vi "Main_25A.vi"() -> ()   [LabVIEW 2024]
uses:
  Utility/Universal Utility/TypeDefs_Utility/Cluster_Row-Column.ctl
  9e3f57c0-2ef8-4495-8287-c6a42a5fb955.vi
  Utility/Universal Utility/TypeDefs_Utility/ENUM_4 Directions U-D-L-R.ctl
  Utility/Universal Utility/TypeDefs_Utility/ENUM_8 Directions U-D-L-R.ctl
panel:
  out "Keys":u32[][](array[numeric])
  out "Locks":u32[][](array[numeric])
  in  "Select Data":enum32{"Example", "Puzzle"}(tab)
  in  "Example":string="#####\n.####\n.####\n.####\n.#.#.\n.#...\n.....\n\n#####\n##.##\n.#.##\n...##\n...#.\n...#.\n.....\n\n.....\n#....\n#....\n#...#\n#.#.#\n#.###\n#####\n\n.....\n.....\n#.#..\n###..\n###.#\n###.#\n#####\n\n.....\n.....\n.....\n#....\n#.#..\n#.#.#\n#####"
  in  "Puzzle":string=".....\n..#..\n..#.#\n..#.#\n#.###\n#####\n#####\n\n#####\n.#.##\n.#..#\n.....\n.....\n.....\n.....\n\n.....\n.....\n.....\n....#\n.#.##\n##.##\n#####\n\n.....\n.....\n.....\n#..#.\n#..##\n#.###\n#####\n\n.....\n#....\n#.#..\n###..\n####.\n#####\n#####\n\n.....\n#....\n#....\n#.#.#\n#.#.#\n#.#.#\n#####\n\n#####\n#.#.#\n....#\n....#\n....#\n.....\n.....\n\n#####\n.####\n.##.#\n.##..\n.##..\n..#..\n.....\n\n#####\n#.###\n#.###\n#.###\n#..#.\n.....\n.....\n\n#####\n#.###\n#.###\n#.#.#\n#.#.#\n.....\n.....\n\n.....\n..#..\n#.#..\n###..\n####.\n####.\n#####\n\n.....\n#....\n#.#..\n#.#..\n####.\n####.\n#####\n\n#####\n.###.\n..#..\n..#..\n..#..\n.....\n.....\n\n.....\n....#\n..#.#\n.##.#\n.##.#\n.##.#\n#####\n\n.....\n.....\n..#..\n..##.\n.###.\n.###.\n#####\n\n.....\n.....\n.....\n.#..#\n###.#\n#####\n#####\n\n#####\n##.##\n##.#.\n##.#.\n##...\n.#...\n.....\n\n#####\n#####\n#.###\n#.#.#\n#...#\n#....\n.....\n\n#####\n.#.##\n...##\n....#\n....#\n....#\n.....\n\n.....\n#....\n##..#\n##.##\n##.##\n##.##\n#####\n\n.....\n.....\n#....\n#...#\n#.#.#\n#.#.#\n#####\n\n#####\n.#.##\n.#.#.\n.#...\n.#...\n.#...\n.....\n\n.....\n#....\n##..#\n###.#\n###.#\n###.#\n#####\n\n#####\n###.#\n#.#.#\n#.#.#\n#...#\n#...#\n.....\n\n#####\n##.#.\n##.#.\n.#.#.\n.#...\n.....\n.....\n\n#####\n#####\n.##.#\n.##..\n.#...\n.#...\n.....\n\n#####\n#####\n#.###\n#.###\n#..#.\n#..#.\n.....\n\n.....\n#....\n##...\n##.#.\n####.\n####.\n#####\n\n.....\n....#\n.#.##\n.#.##\n.####\n#####\n#####\n\n.....\n#....\n#.#.#\n#.#.#\n#####\n#####\n#####\n\n#####\n####.\n####.\n#.##.\n..##.\n..#..\n.....\n\n.....\n#....\n##...\n##...\n##.#.\n##.#.\n#####\n\n.....\n.#..#\n.##.#\n.####\n#####\n#####\n#####\n\n.....\n...#.\n...#.\n.#.#.\n#####\n#####\n#####\n\n.....\n.....\n...#.\n..##.\n#.##.\n#####\n#####\n\n#####\n##.#.\n.#.#.\n.#.#.\n.#.#.\n...#.\n.....\n\n#####\n#.#.#\n..#.#\n..#.#\n.....\n.....\n.....\n\n#####\n#####\n.###.\n.###.\n.###.\n.#.#.\n.....\n\n.....\n.....\n..#..\n..#..\n.##.#\n.####\n#####\n\n#####\n#.###\n#.###\n...#.\n...#.\n.....\n.....\n\n.....\n.....\n.#...\n.##..\n.###.\n####.\n#####\n\n.....\n#.#.#\n#.#.#\n###.#\n###.#\n###.#\n#####\n\n#####\n#####\n#####\n#####\n#.##.\n#.#..\n.....\n\n.....\n.....\n..#..\n..#..\n#.#..\n###.#\n#####\n\n#####\n#####\n###.#\n###..\n#.#..\n#.#..\n.....\n\n#####\n#####\n##.##\n#..#.\n#..#.\n#....\n.....\n\n.....\n..#..\n.##..\n###.#\n###.#\n###.#\n#####\n\n.....\n.#...\n.#...\n.#.#.\n.#.##\n.####\n#####\n\n.....\n.#...\n###..\n###.#\n###.#\n###.#\n#####\n\n.....\n...#.\n#.##.\n#####\n#####\n#####\n#####\n\n.....\n...#.\n...#.\n#..#.\n#..#.\n##.#.\n#####\n\n#####\n.####\n.###.\n.#.#.\n.....\n.....\n.....\n\n.....\n#.#..\n#.#.#\n#.###\n#.###\n#####\n#####\n\n#####\n#####\n###.#\n#.#..\n#.#..\n.....\n.....\n\n.....\n#.#..\n#.##.\n####.\n####.\n####.\n#####\n\n#####\n#####\n##.##\n#..#.\n#..#.\n#..#.\n.....\n\n.....\n#.#.#\n#.#.#\n#.#.#\n###.#\n###.#\n#####\n\n#####\n#####\n#####\n####.\n#.##.\n..#..\n.....\n\n.....\n.....\n....#\n....#\n..#.#\n#.#.#\n#####\n\n.....\n..#.#\n#.#.#\n#.#.#\n#.###\n#.###\n#####\n\n#####\n#.##.\n...#.\n...#.\n...#.\n...#.\n.....\n\n.....\n...#.\n.#.##\n#####\n#####\n#####\n#####\n\n#####\n##.##\n##.#.\n##.#.\n#....\n.....\n.....\n\n.....\n..#..\n..#.#\n..###\n.####\n#####\n#####\n\n#####\n####.\n####.\n####.\n##.#.\n.#.#.\n.....\n\n#####\n#####\n###.#\n#.#..\n..#..\n.....\n.....\n\n.....\n#....\n#....\n#...#\n#.#.#\n#.###\n#####\n\n.....\n.....\n#.#.#\n#.#.#\n#.#.#\n#.###\n#####\n\n#####\n.####\n..###\n..#.#\n....#\n.....\n.....\n\n.....\n#...#\n#...#\n#.#.#\n#.#.#\n#.#.#\n#####\n\n#####\n###.#\n###..\n.##..\n..#..\n.....\n.....\n\n.....\n.....\n#..#.\n##.#.\n##.#.\n#####\n#####\n\n.....\n..#..\n..##.\n..##.\n..###\n#.###\n#####\n\n#####\n.##.#\n.#...\n.#...\n.#...\n.#...\n.....\n\n#####\n##.##\n##.##\n.#..#\n.#..#\n.....\n.....\n\n.....\n....#\n#...#\n#...#\n#...#\n#.#.#\n#####\n\n.....\n.....\n#....\n#..#.\n##.#.\n##.##\n#####\n\n.....\n.....\n...#.\n.#.#.\n.#.#.\n####.\n#####\n\n#####\n.####\n..##.\n..##.\n..##.\n...#.\n.....\n\n#####\n#.#.#\n..#.#\n..#.#\n..#.#\n..#.#\n.....\n\n#####\n.#.##\n.#.##\n...##\n....#\n.....\n.....\n\n.....\n#...#\n#...#\n##.##\n##.##\n#####\n#####\n\n#####\n#####\n####.\n.###.\n.#.#.\n.....\n.....\n\n#####\n#####\n###.#\n.##.#\n.#..#\n.#...\n.....\n\n#####\n##.##\n##.##\n##..#\n##..#\n.#...\n.....\n\n#####\n#####\n#####\n##.##\n#..##\n...#.\n.....\n\n#####\n#.###\n#.###\n#.#.#\n#.#..\n#.#..\n.....\n\n.....\n....#\n..#.#\n#.#.#\n#.#.#\n#.###\n#####\n\n.....\n.#...\n.#.#.\n.#.##\n.####\n#####\n#####\n\n#####\n#.##.\n#.##.\n#.#..\n#.#..\n#.#..\n.....\n\n.....\n.....\n.....\n#....\n##.#.\n##.##\n#####\n\n.....\n..#..\n..##.\n..##.\n.####\n#####\n#####\n\n#####\n#.##.\n#.#..\n#.#..\n..#..\n..#..\n.....\n\n.....\n.#..#\n.#..#\n.#.##\n##.##\n##.##\n#####\n\n.....\n.....\n....#\n#.#.#\n#.#.#\n#####\n#####\n\n.....\n.....\n...#.\n.#.##\n.#.##\n.#.##\n#####\n\n#####\n###.#\n.##.#\n.#...\n.#...\n.....\n.....\n\n.....\n..#..\n..#..\n..##.\n.####\n.####\n#####\n\n#####\n#.###\n..##.\n..##.\n..#..\n..#..\n.....\n\n#####\n.####\n..###\n..###\n...#.\n.....\n.....\n\n#####\n#.##.\n..##.\n..##.\n...#.\n...#.\n.....\n\n#####\n#.#.#\n#...#\n.....\n.....\n.....\n.....\n\n.....\n..#..\n..#.#\n#.#.#\n#.#.#\n#.#.#\n#####\n\n#####\n#####\n.###.\n.#.#.\n.#...\n.....\n.....\n\n#####\n#####\n#####\n#.#.#\n..#..\n..#..\n.....\n\n.....\n...#.\n...#.\n..##.\n.####\n#####\n#####\n\n#####\n###.#\n###..\n#.#..\n.....\n.....\n.....\n\n.....\n.....\n.#.#.\n.#.#.\n##.##\n#####\n#####\n\n.....\n.....\n..#.#\n#.#.#\n###.#\n#####\n#####\n\n.....\n.#...\n.#..#\n##..#\n##..#\n###.#\n#####\n\n#####\n#####\n#####\n#.##.\n#.##.\n..#..\n.....\n\n.....\n#..#.\n#..#.\n#.###\n#.###\n#####\n#####\n\n.....\n.....\n.#...\n.#..#\n.#.##\n.####\n#####\n\n.....\n.#.#.\n####.\n####.\n#####\n#####\n#####\n\n#####\n#.###\n#.##.\n..##.\n..##.\n..#..\n.....\n\n.....\n..#..\n..#.#\n..###\n#.###\n#####\n#####\n\n.....\n.....\n.....\n.#..#\n###.#\n###.#\n#####\n\n#####\n#####\n#####\n####.\n#.#..\n.....\n.....\n\n.....\n.....\n...#.\n...##\n.#.##\n#####\n#####\n\n.....\n.#...\n.#...\n.#...\n##...\n###.#\n#####\n\n.....\n..#.#\n..#.#\n#.#.#\n#####\n#####\n#####\n\n#####\n#####\n##.##\n##.##\n#...#\n#....\n.....\n\n.....\n....#\n#...#\n#...#\n#.#.#\n###.#\n#####\n\n.....\n....#\n....#\n..#.#\n..#.#\n.##.#\n#####\n\n#####\n####.\n.#.#.\n.#.#.\n.#.#.\n.#.#.\n.....\n\n#####\n#.#.#\n#.#.#\n#.#.#\n#.#.#\n#.#.#\n.....\n\n#####\n###.#\n##..#\n##..#\n##..#\n#...#\n.....\n\n#####\n#.###\n#.#.#\n#...#\n#...#\n#....\n.....\n\n#####\n#####\n###.#\n##..#\n.#..#\n.#..#\n.....\n\n.....\n.....\n.....\n#....\n#.#..\n#.##.\n#####\n\n#####\n.####\n.##.#\n..#.#\n..#.#\n....#\n.....\n\n.....\n.....\n..#..\n..#.#\n.##.#\n###.#\n#####\n\n.....\n#..#.\n#.##.\n####.\n####.\n#####\n#####\n\n.....\n..#..\n..#..\n#.##.\n#.###\n#####\n#####\n\n#####\n#####\n##.##\n.#.#.\n.#.#.\n...#.\n.....\n\n#####\n##.##\n##.##\n#...#\n#....\n#....\n.....\n\n.....\n.....\n.....\n..#.#\n..###\n.####\n#####\n\n.....\n#.#..\n#.##.\n#.###\n#.###\n#####\n#####\n\n.....\n#....\n#...#\n##.##\n##.##\n#####\n#####\n\n#####\n####.\n#.##.\n..##.\n..##.\n...#.\n.....\n\n#####\n#.##.\n#.##.\n#.##.\n..#..\n..#..\n.....\n\n#####\n##.##\n##.##\n##.##\n.#.##\n.#.#.\n.....\n\n#####\n#####\n#####\n#.#.#\n#.#.#\n#....\n.....\n\n#####\n####.\n.###.\n.###.\n..#..\n.....\n.....\n\n.....\n.#..#\n.#.##\n.#.##\n.#.##\n.#.##\n#####\n\n#####\n.####\n.####\n.###.\n.#.#.\n.#.#.\n.....\n\n.....\n.....\n.#...\n.##..\n###.#\n###.#\n#####\n\n.....\n.....\n....#\n....#\n#.#.#\n#####\n#####\n\n#####\n#####\n##.##\n#..#.\n#..#.\n...#.\n.....\n\n#####\n.####\n..###\n...#.\n...#.\n...#.\n.....\n\n.....\n....#\n.#.##\n.#.##\n.#.##\n.#.##\n#####\n\n.....\n#....\n#..#.\n##.#.\n##.#.\n##.#.\n#####\n\n.....\n...#.\n...#.\n#.##.\n#.##.\n#.##.\n#####\n\n.....\n.#..#\n.##.#\n#####\n#####\n#####\n#####\n\n#####\n.###.\n..##.\n..#..\n..#..\n..#..\n.....\n\n#####\n#.#.#\n#.#.#\n..#.#\n..#.#\n....#\n.....\n\n#####\n#####\n##.#.\n##.#.\n##...\n#....\n.....\n\n#####\n#####\n##.#.\n.#.#.\n...#.\n...#.\n.....\n\n#####\n.####\n.#.##\n.#..#\n.#..#\n.#...\n.....\n\n#####\n#####\n###.#\n.##.#\n.#...\n.....\n.....\n\n#####\n#####\n###.#\n.##.#\n.##.#\n..#.#\n.....\n\n#####\n#.###\n..###\n..###\n...##\n...#.\n.....\n\n.....\n.#...\n.#...\n.##.#\n###.#\n###.#\n#####\n\n#####\n#####\n#####\n#####\n##.##\n.#..#\n.....\n\n.....\n#....\n#...#\n#.#.#\n###.#\n###.#\n#####\n\n#####\n.#.##\n.#..#\n.#...\n.....\n.....\n.....\n\n.....\n..#..\n#.##.\n#.##.\n#.##.\n####.\n#####\n\n#####\n##.#.\n##.#.\n##...\n.#...\n.#...\n.....\n\n.....\n.....\n.#...\n###.#\n###.#\n#####\n#####\n\n#####\n#####\n#####\n###.#\n.##.#\n.#..#\n.....\n\n.....\n..#..\n.##..\n.##..\n.###.\n.###.\n#####\n\n#####\n#####\n#####\n#.##.\n...#.\n...#.\n.....\n\n.....\n#...#\n##.##\n##.##\n##.##\n#####\n#####\n\n.....\n.....\n..#..\n.##..\n.##.#\n.####\n#####\n\n.....\n.....\n....#\n#.#.#\n#.#.#\n#.###\n#####\n\n#####\n#####\n#####\n#####\n.#.#.\n.....\n.....\n\n#####\n##.##\n.#..#\n.#..#\n....#\n....#\n.....\n\n.....\n..#..\n#.#..\n#.##.\n#.##.\n####.\n#####\n\n.....\n.....\n.#...\n.##..\n.##.#\n.##.#\n#####\n\n.....\n.....\n.#...\n.#...\n.##.#\n#####\n#####\n\n.....\n#...#\n##.##\n##.##\n#####\n#####\n#####\n\n.....\n#.#..\n####.\n#####\n#####\n#####\n#####\n\n.....\n..#.#\n..#.#\n.##.#\n.##.#\n###.#\n#####\n\n#####\n####.\n##.#.\n##...\n.#...\n.#...\n.....\n\n#####\n#####\n###.#\n###.#\n#.#.#\n..#.#\n.....\n\n#####\n#####\n#####\n.####\n..#.#\n.....\n.....\n\n.....\n...#.\n.#.#.\n.#.##\n##.##\n##.##\n#####\n\n.....\n.....\n..#..\n..#.#\n..###\n.####\n#####\n\n#####\n#.###\n#.#.#\n#.#..\n..#..\n.....\n.....\n\n.....\n....#\n..#.#\n..###\n..###\n#.###\n#####\n\n#####\n#.###\n#.#.#\n#.#..\n..#..\n..#..\n.....\n\n#####\n#####\n#####\n#.###\n#.##.\n#..#.\n.....\n\n.....\n.#...\n.#.#.\n.#.#.\n##.##\n##.##\n#####\n\n#####\n.#.#.\n.#.#.\n...#.\n...#.\n.....\n.....\n\n.....\n...#.\n..##.\n..##.\n#.###\n#.###\n#####\n\n.....\n#....\n#..#.\n#..#.\n##.##\n#####\n#####\n\n#####\n#####\n.###.\n..#..\n..#..\n.....\n.....\n\n#####\n#####\n###.#\n#.#.#\n..#..\n..#..\n.....\n\n.....\n.#...\n.#.#.\n.#.#.\n##.#.\n#####\n#####\n\n.....\n.#...\n##...\n##...\n###.#\n###.#\n#####\n\n.....\n.....\n...#.\n#..##\n#.###\n#####\n#####\n\n.....\n.....\n#....\n##.#.\n##.#.\n#####\n#####\n\n.....\n.....\n...#.\n..##.\n#.##.\n####.\n#####\n\n#####\n#.#.#\n#.#.#\n#.#..\n#.#..\n.....\n.....\n\n.....\n#.#..\n###..\n####.\n####.\n#####\n#####\n\n.....\n.....\n.#..#\n.#..#\n.#..#\n.#.##\n#####\n\n#####\n.####\n.###.\n..#..\n..#..\n.....\n.....\n\n#####\n#.###\n#.##.\n#.##.\n..##.\n...#.\n.....\n\n#####\n##.##\n.#.##\n.#..#\n....#\n....#\n.....\n\n#####\n##.##\n##.##\n##.#.\n.#...\n.....\n.....\n\n.....\n#..#.\n##.#.\n##.#.\n##.#.\n####.\n#####\n\n.....\n.#...\n.#...\n.#.#.\n.#.#.\n##.##\n#####\n\n.....\n.....\n.....\n..#..\n..#..\n#.##.\n#####\n\n#####\n##.##\n.#.##\n.#.##\n.#.#.\n...#.\n.....\n\n.....\n#....\n#....\n##...\n###.#\n###.#\n#####\n\n.....\n.#..#\n.#..#\n##..#\n##..#\n###.#\n#####\n\n.....\n.....\n.....\n#...#\n#.#.#\n#.#.#\n#####\n\n#####\n####.\n####.\n####.\n#.##.\n..#..\n.....\n\n#####\n##.#.\n##.#.\n.#.#.\n.#.#.\n.#.#.\n.....\n\n.....\n.....\n..#.#\n.##.#\n.##.#\n.##.#\n#####\n\n#####\n#####\n####.\n.###.\n.#.#.\n.#...\n.....\n\n.....\n.....\n.....\n...#.\n..##.\n#.###\n#####\n\n#####\n####.\n#.##.\n..#..\n..#..\n.....\n.....\n\n.....\n.....\n..#..\n#.#..\n#.#.#\n#.###\n#####\n\n#####\n#.#.#\n#...#\n#....\n#....\n.....\n.....\n\n.....\n#...#\n#..##\n##.##\n#####\n#####\n#####\n\n#####\n#.##.\n#.##.\n#.#..\n#.#..\n..#..\n.....\n\n.....\n.#...\n.#..#\n.#..#\n.#.##\n#####\n#####\n\n.....\n.....\n#.#..\n#.##.\n#.##.\n#.###\n#####\n\n#####\n###.#\n.##.#\n.#..#\n.#...\n.#...\n.....\n\n.....\n..#..\n..#.#\n..###\n..###\n#.###\n#####\n\n.....\n#...#\n#...#\n#..##\n#.###\n#.###\n#####\n\n.....\n#.#..\n#.#..\n#.#..\n#.##.\n####.\n#####\n\n#####\n.####\n.###.\n.#.#.\n.#.#.\n.#.#.\n.....\n\n#####\n##.##\n.#.##\n...##\n...##\n....#\n.....\n\n#####\n.###.\n.##..\n..#..\n..#..\n.....\n.....\n\n#####\n##.#.\n##.#.\n#..#.\n...#.\n...#.\n.....\n\n#####\n#.###\n#.###\n#.#.#\n#.#..\n..#..\n.....\n\n.....\n#..#.\n#.##.\n#.###\n#.###\n#.###\n#####\n\n.....\n.....\n#.#..\n#.#..\n###..\n####.\n#####\n\n.....\n#....\n#...#\n#.#.#\n#####\n#####\n#####\n\n.....\n....#\n#.#.#\n#.#.#\n###.#\n#####\n#####\n\n#####\n.####\n.####\n..#.#\n....#\n.....\n.....\n\n.....\n.....\n#..#.\n#..##\n##.##\n##.##\n#####\n\n#####\n#.###\n...##\n...#.\n...#.\n.....\n.....\n\n.....\n.....\n....#\n.#..#\n##..#\n##.##\n#####\n\n#####\n#####\n#####\n#####\n.#.##\n.#..#\n.....\n\n#####\n#####\n#####\n####.\n#.#..\n..#..\n.....\n\n.....\n.#...\n.#.#.\n.#.#.\n.#.#.\n.#.#.\n#####\n\n#####\n#.###\n#.###\n#.#.#\n#.#..\n#....\n.....\n\n.....\n...#.\n...#.\n.#.##\n#####\n#####\n#####\n\n#####\n.####\n..###\n..###\n..#.#\n..#..\n.....\n\n#####\n#####\n#####\n#####\n##.##\n.#.#.\n.....\n\n#####\n.####\n.##.#\n..#.#\n.....\n.....\n.....\n\n#####\n#####\n#.###\n#..##\n#..##\n....#\n.....\n\n.....\n.#..#\n###.#\n###.#\n###.#\n#####\n#####\n\n.....\n...#.\n...#.\n#..##\n##.##\n#####\n#####\n\n#####\n#.##.\n#.#..\n#.#..\n#....\n.....\n.....\n\n#####\n###.#\n###.#\n##..#\n#...#\n.....\n.....\n\n#####\n#####\n#.###\n#.##.\n#.#..\n#....\n.....\n\n.....\n.....\n..#..\n#.#..\n#.#.#\n###.#\n#####\n\n#####\n##.##\n#..##\n...#.\n...#.\n.....\n.....\n\n.....\n..#..\n..#..\n.##..\n.##..\n.##.#\n#####\n\n#####\n#####\n.####\n.#.##\n...##\n....#\n.....\n\n#####\n.####\n.####\n..###\n...#.\n.....\n.....\n\n#####\n#####\n#.##.\n#.##.\n#..#.\n.....\n.....\n\n#####\n#.#.#\n#.#..\n#.#..\n.....\n.....\n.....\n\n.....\n.....\n..#..\n..#..\n..##.\n.####\n#####\n\n#####\n###.#\n##..#\n.#..#\n.#..#\n.#..#\n.....\n\n#####\n###.#\n###.#\n#.#..\n.....\n.....\n.....\n\n#####\n#.##.\n#..#.\n#....\n.....\n.....\n.....\n\n.....\n.....\n.....\n.....\n#..#.\n#.##.\n#####\n\n#####\n####.\n##.#.\n#..#.\n#..#.\n...#.\n.....\n\n.....\n..#..\n.##.#\n###.#\n###.#\n#####\n#####\n\n.....\n.#...\n.#.#.\n.###.\n.###.\n#####\n#####\n\n#####\n#.##.\n#..#.\n.....\n.....\n.....\n.....\n\n.....\n#....\n#..#.\n##.#.\n##.##\n#####\n#####\n\n#####\n#.###\n#.#.#\n#....\n#....\n.....\n.....\n\n#####\n#####\n##.#.\n##.#.\n##...\n.#...\n.....\n\n.....\n....#\n..#.#\n..#.#\n..###\n.####\n#####\n\n.....\n..#..\n..#.#\n..#.#\n#.###\n#.###\n#####\n\n#####\n##.##\n.#.##\n.#.##\n...##\n...#.\n.....\n\n#####\n###.#\n##...\n.#...\n.#...\n.....\n.....\n\n#####\n#####\n##.##\n##.#.\n##.#.\n#..#.\n.....\n\n.....\n...#.\n#..#.\n##.#.\n##.#.\n####.\n#####\n\n#####\n.#.#.\n...#.\n...#.\n...#.\n.....\n.....\n\n.....\n.....\n#....\n#....\n#..#.\n#.##.\n#####\n\n.....\n....#\n....#\n#..##\n#.###\n#.###\n#####\n\n#####\n#.###\n#.###\n#.#.#\n#...#\n....#\n.....\n\n#####\n#####\n.####\n.###.\n.#.#.\n.#...\n.....\n\n#####\n####.\n.###.\n..#..\n..#..\n..#..\n.....\n\n.....\n.....\n..#..\n..#.#\n.##.#\n#####\n#####\n\n.....\n.....\n..#.#\n..###\n..###\n#.###\n#####\n\n.....\n#....\n#...#\n##..#\n##..#\n###.#\n#####\n\n#####\n##.##\n##.##\n##..#\n#...#\n#...#\n.....\n\n#####\n##.#.\n.#.#.\n.#.#.\n.#.#.\n.#...\n.....\n\n#####\n####.\n###..\n#.#..\n#.#..\n#.#..\n.....\n\n#####\n##.##\n#..#.\n...#.\n.....\n.....\n.....\n\n#####\n.###.\n.#.#.\n.#.#.\n...#.\n...#.\n.....\n\n.....\n.....\n..#.#\n..#.#\n.##.#\n.##.#\n#####\n\n#####\n#.##.\n#.##.\n#.##.\n#.#..\n.....\n.....\n\n#####\n##.##\n##..#\n##...\n##...\n.#...\n.....\n\n#####\n.####\n.#.##\n.#.##\n.#..#\n....#\n.....\n\n#####\n.###.\n.#.#.\n...#.\n.....\n.....\n.....\n\n.....\n.....\n.#..#\n.##.#\n.##.#\n###.#\n#####\n\n.....\n#....\n#..#.\n#.##.\n#####\n#####\n#####\n\n.....\n#.#..\n#.#..\n#.##.\n####.\n####.\n#####\n\n#####\n#####\n#####\n.###.\n.#.#.\n.#...\n.....\n\n#####\n#####\n#.###\n#.###\n...#.\n...#.\n.....\n\n.....\n.....\n.....\n.....\n.#...\n.#.#.\n#####\n\n.....\n..#..\n..#..\n.###.\n.####\n.####\n#####\n\n#####\n##.##\n##.##\n##.##\n#..##\n#..#.\n.....\n\n#####\n.####\n.#.##\n.#.#.\n.#...\n.#...\n.....\n\n.....\n..#..\n..#..\n.##..\n.###.\n.###.\n#####\n\n#####\n#####\n##.##\n##.##\n##.#.\n.#.#.\n.....\n\n#####\n##.##\n##.##\n#..##\n#...#\n#....\n.....\n\n.....\n.....\n.....\n.#...\n.##.#\n.##.#\n#####\n\n.....\n.#...\n.#...\n.#.#.\n.###.\n.###.\n#####\n\n.....\n.#...\n.#.#.\n##.##\n##.##\n#####\n#####\n\n#####\n#####\n#.##.\n#..#.\n#..#.\n#..#.\n.....\n\n#####\n.####\n.##.#\n.##.#\n..#.#\n.....\n.....\n\n#####\n#####\n#.###\n#.#.#\n....#\n.....\n.....\n\n.....\n..#.#\n..###\n#.###\n#####\n#####\n#####\n\n#####\n###.#\n.##.#\n.##..\n.##..\n.#...\n.....\n\n.....\n.#...\n.##..\n###.#\n#####\n#####\n#####\n\n.....\n.#...\n.#...\n.#.#.\n.#.##\n#####\n#####\n\n#####\n.####\n.###.\n..#..\n..#..\n..#..\n.....\n\n.....\n.#...\n.#...\n.#.#.\n.#.#.\n.####\n#####\n\n.....\n.#..#\n.#..#\n.#.##\n.#.##\n.#.##\n#####\n\n#####\n##.#.\n.#...\n.#...\n.....\n.....\n.....\n\n#####\n#####\n#####\n##.##\n#..#.\n#....\n.....\n\n#####\n#####\n#.#.#\n#.#..\n..#..\n.....\n.....\n\n#####\n#.#.#\n#.#.#\n#.#.#\n#.#..\n.....\n.....\n\n.....\n#....\n#....\n##...\n##.#.\n####.\n#####\n\n.....\n.....\n#.#..\n#.#.#\n#.###\n#.###\n#####\n\n#####\n###.#\n##..#\n##..#\n##...\n.#...\n.....\n\n.....\n.....\n#..#.\n#..#.\n#.##.\n#.###\n#####\n\n#####\n#####\n###.#\n#.#.#\n#.#.#\n..#.#\n.....\n\n.....\n...#.\n#..#.\n#..##\n#..##\n##.##\n#####\n\n.....\n....#\n#.#.#\n#.#.#\n#.#.#\n###.#\n#####\n\n.....\n.....\n.....\n....#\n.#..#\n.#.##\n#####\n\n.....\n.#.#.\n####.\n#####\n#####\n#####\n#####\n\n.....\n.....\n.....\n.....\n#.#.#\n#.###\n#####\n\n.....\n.#.#.\n.###.\n.####\n#####\n#####\n#####\n\n#####\n#.###\n#..##\n#..#.\n...#.\n...#.\n.....\n\n#####\n#####\n###.#\n##..#\n.#..#\n.#...\n.....\n\n.....\n.....\n...#.\n.#.##\n##.##\n##.##\n#####\n\n.....\n..#..\n#.#..\n###..\n###..\n###.#\n#####\n\n.....\n#....\n#....\n#..#.\n#.##.\n#.###\n#####\n\n#####\n#####\n#####\n#.##.\n#..#.\n...#.\n.....\n\n#####\n#####\n.####\n.####\n.##.#\n.#...\n.....\n\n.....\n.#.#.\n.#.#.\n.#.#.\n##.##\n#####\n#####\n\n.....\n#....\n#..#.\n##.#.\n####.\n#####\n#####\n\n#####\n#.###\n#.#.#\n..#.#\n..#.#\n.....\n.....\n\n#####\n###.#\n###..\n###..\n##...\n#....\n.....\n\n.....\n...#.\n#..#.\n#..##\n#.###\n#.###\n#####\n\n.....\n.....\n#..#.\n#..##\n#..##\n##.##\n#####\n\n.....\n....#\n....#\n.#..#\n.#..#\n##.##\n#####\n\n#####\n####.\n##.#.\n##.#.\n##.#.\n#..#.\n.....\n\n#####\n##.##\n.#..#\n.#..#\n.#..#\n....#\n.....\n\n#####\n#.###\n#.###\n..##.\n..#..\n.....\n.....\n\n.....\n...#.\n...#.\n...#.\n.#.##\n.#.##\n#####\n\n.....\n.#...\n.#...\n###..\n###.#\n#####\n#####\n\n#####\n##.##\n.#..#\n....#\n....#\n....#\n.....\n\n#####\n##.##\n##.#.\n.#...\n.#...\n.....\n.....\n\n#####\n##.##\n#..##\n#..##\n#..##\n#...#\n.....\n\n.....\n..#..\n#.#..\n###..\n####.\n#####\n#####\n\n.....\n#.#.#\n###.#\n###.#\n###.#\n###.#\n#####\n\n#####\n.####\n.####\n.####\n.#.#.\n.#...\n.....\n\n.....\n.#.#.\n.#.#.\n.#.##\n#####\n#####\n#####\n\n.....\n#...#\n#.#.#\n#.#.#\n#####\n#####\n#####\n\n.....\n.#...\n.#.#.\n.###.\n####.\n####.\n#####\n\n#####\n###.#\n###.#\n###..\n#.#..\n#.#..\n.....\n\n.....\n.....\n.....\n..#..\n..#.#\n#.#.#\n#####\n\n#####\n##.##\n##.#.\n#..#.\n#..#.\n#....\n.....\n\n.....\n...#.\n..###\n..###\n#.###\n#.###\n#####\n\n#####\n####.\n.#.#.\n.#.#.\n.#.#.\n.#...\n.....\n\n#####\n###.#\n#.#.#\n#.#..\n#.#..\n..#..\n.....\n\n#####\n##.##\n##..#\n#...#\n#....\n.....\n.....\n\n#####\n.####\n..###\n..###\n..#.#\n....#\n.....\n\n#####\n.##.#\n..#.#\n..#.#\n..#.#\n..#.#\n.....\n\n#####\n#####\n.####\n.####\n..#.#\n..#..\n.....\n\n#####\n#.###\n#..#.\n.....\n.....\n.....\n.....\n\n.....\n.....\n..#.#\n..#.#\n..#.#\n.##.#\n#####\n\n#####\n#####\n##.##\n##.##\n.#.#.\n...#.\n.....\n\n#####\n##.##\n#..##\n#..##\n#..#.\n.....\n.....\n\n#####\n.####\n.#.#.\n.#...\n.....\n.....\n.....\n\n.....\n.#...\n.#...\n.#..#\n.#.##\n.####\n#####\n\n.....\n#....\n#...#\n#.#.#\n###.#\n#####\n#####\n\n.....\n....#\n#.#.#\n#.#.#\n#.#.#\n#.###\n#####\n\n#####\n####.\n.##..\n..#..\n.....\n.....\n.....\n\n#####\n#####\n#####\n###.#\n##...\n.#...\n.....\n\n#####\n#####\n##.##\n#..#.\n#..#.\n.....\n.....\n\n#####\n#####\n#####\n##.#.\n##.#.\n#....\n.....\n\n.....\n#..#.\n#.##.\n#.##.\n#####\n#####\n#####\n\n#####\n#####\n.####\n..#.#\n....#\n.....\n.....\n\n#####\n#.#.#\n..#.#\n..#..\n..#..\n.....\n.....\n\n#####\n##.#.\n##.#.\n##...\n#....\n.....\n.....\n\n.....\n..#.#\n..#.#\n.####\n.####\n#####\n#####\n\n.....\n#....\n#....\n##...\n###.#\n#####\n#####\n\n#####\n##.#.\n##.#.\n.#.#.\n.#.#.\n.#...\n.....\n\n.....\n.#...\n##..#\n##..#\n###.#\n###.#\n#####\n\n.....\n#...#\n##.##\n##.##\n##.##\n##.##\n#####\n\n.....\n.#...\n.#...\n.#...\n.##.#\n###.#\n#####\n\n.....\n....#\n.#.##\n.#.##\n.####\n.####\n#####\n\n.....\n.#...\n##..#\n##.##\n##.##\n##.##\n#####\n\n.....\n.....\n.....\n....#\n.#..#\n##.##\n#####\n\n.....\n.#.#.\n##.#.\n##.#.\n##.#.\n####.\n#####\n\n#####\n#####\n###.#\n###.#\n#.#.#\n..#..\n.....\n\n.....\n..#..\n..#..\n..##.\n..##.\n#.##.\n#####\n\n.....\n.....\n.....\n....#\n.#.##\n.####\n#####\n\n.....\n.#.#.\n.#.#.\n.#.#.\n.###.\n.###.\n#####\n\n#####\n##.##\n##.##\n##..#\n#...#\n#....\n.....\n\n#####\n###.#\n.#...\n.....\n.....\n.....\n.....\n\n#####\n#.###\n#.#.#\n#.#.#\n#...#\n#...#\n.....\n\n#####\n###.#\n.##..\n.##..\n.##..\n..#..\n.....\n\n#####\n####.\n####.\n###..\n.#...\n.#...\n.....\n\n#####\n####.\n#.#..\n#.#..\n#....\n.....\n.....\n\n#####\n.#.##\n.#.##\n.#.##\n.#..#\n.#..#\n.....\n\n#####\n#.###\n#..##\n#..#.\n.....\n.....\n.....\n\n#####\n#####\n#.###\n#.##.\n#.#..\n#.#..\n.....\n\n#####\n.##.#\n.#..#\n.#..#\n....#\n.....\n.....\n\n#####\n#####\n#.##.\n#.##.\n#.##.\n..#..\n.....\n\n.....\n.....\n...#.\n.#.#.\n.#.#.\n##.#.\n#####\n\n.....\n...#.\n...#.\n...##\n..###\n.####\n#####\n\n#####\n#####\n#####\n###.#\n.##..\n.#...\n.....\n\n#####\n#####\n##.##\n#...#\n#....\n#....\n.....\n\n#####\n####.\n.###.\n.#.#.\n...#.\n.....\n.....\n\n.....\n.....\n.....\n..#..\n.##..\n.###.\n#####\n\n#####\n###.#\n##...\n##...\n.#...\n.....\n.....\n\n.....\n..#..\n..#..\n.###.\n.####\n#####\n#####\n\n#####\n.###.\n.##..\n.##..\n.#...\n.#...\n.....\n\n.....\n....#\n#...#\n#...#\n##.##\n##.##\n#####\n\n#####\n##.##\n.#.#.\n.#.#.\n.....\n.....\n.....\n\n#####\n#.###\n#.###\n#.###\n#..##\n...#.\n.....\n\n#####\n.##.#\n.#..#\n....#\n....#\n....#\n.....\n\n.....\n.....\n.#...\n.#.#.\n.####\n.####\n#####\n\n.....\n#....\n#.#..\n#.##.\n####.\n#####\n#####\n\n#####\n##.#.\n##.#.\n##.#.\n##...\n#....\n.....\n\n.....\n.#.#.\n##.#.\n##.#.\n##.##\n#####\n#####\n\n.....\n.#.#.\n.#.#.\n.#.##\n.####\n#####\n#####\n\n.....\n.#...\n##.#.\n##.##\n##.##\n#####\n#####\n\n.....\n.....\n.#...\n.#.#.\n####.\n####.\n#####\n\n.....\n....#\n.#..#\n##.##\n##.##\n##.##\n#####\n\n#####\n#####\n#####\n#.#.#\n#.#.#\n..#..\n.....\n\n.....\n#...#\n#...#\n##.##\n##.##\n##.##\n#####\n\n.....\n.....\n#...#\n#.#.#\n#.###\n#.###\n#####\n\n#####\n.####\n.####\n.#.#.\n.....\n.....\n.....\n\n.....\n.#...\n##...\n##..#\n##.##\n#####\n#####\n\n#####\n.####\n.#.##\n.#..#\n.....\n.....\n.....\n\n#####\n.####\n.##.#\n.##.#\n.#..#\n.#...\n.....\n\n.....\n.....\n.....\n.....\n#.#..\n#.#.#\n#####\n\n.....\n.....\n...#.\n...#.\n.#.#.\n.#.##\n#####\n\n.....\n..#..\n..#..\n#.#..\n#.#..\n#.#.#\n#####\n\n.....\n.....\n.....\n.#.#.\n##.#.\n##.##\n#####\n\n.....\n...#.\n..##.\n#.##.\n#.###\n#####\n#####\n\n#####\n##.##\n##.##\n##.#.\n.#...\n.#...\n.....\n\n.....\n.....\n#....\n#.#..\n#.#..\n####.\n#####\n\n.....\n.....\n...#.\n.#.#.\n##.##\n##.##\n#####\n\n.....\n.....\n.#..#\n.##.#\n.##.#\n#####\n#####\n\n.....\n..#..\n.##..\n.##..\n.##.#\n.####\n#####\n\n.....\n.#..#\n.##.#\n.##.#\n#####\n#####\n#####\n\n.....\n.....\n#..#.\n#.###\n#.###\n#.###\n#####\n\n.....\n.#.#.\n.#.#.\n##.#.\n##.#.\n##.#.\n#####\n\n#####\n###.#\n#.#..\n#....\n.....\n.....\n.....\n\n#####\n#####\n.#.##\n.#.##\n.#.##\n....#\n.....\n\n#####\n#.###\n#.#.#\n#...#\n....#\n.....\n.....\n\n#####\n###.#\n.##.#\n..#.#\n..#.#\n..#.#\n.....\n\n#####\n###.#\n.##.#\n.##..\n..#..\n..#..\n.....\n\n#####\n.##.#\n.##.#\n.#..#\n.....\n.....\n.....\n\n#####\n#####\n.####\n.##.#\n..#..\n.....\n.....\n\n#####\n#.###\n#..##\n...##\n...#.\n.....\n.....\n\n#####\n#####\n#####\n#####\n#.###\n..#.#\n.....\n\n.....\n....#\n.#..#\n.#..#\n.#.##\n#####\n#####\n\n#####\n#####\n#####\n##.##\n##.##\n#...#\n.....\n\n.....\n.....\n.....\n..#..\n.##..\n.##.#\n#####\n\n#####\n#####\n####.\n####.\n.#.#.\n...#.\n.....\n\n.....\n.#..#\n.#.##\n.#.##\n##.##\n#####\n#####\n\n.....\n..#.#\n..#.#\n..#.#\n#.###\n#.###\n#####\n\n#####\n#####\n####.\n##.#.\n#..#.\n#..#.\n.....\n\n.....\n.....\n.....\n.#.#.\n.#.#.\n.###.\n#####\n\n.....\n..#..\n#.#..\n#.#.#\n#####\n#####\n#####\n\n#####\n###.#\n##..#\n.#...\n.#...\n.....\n.....\n\n#####\n#.###\n#.##.\n#.##.\n#.#..\n#....\n.....\n\n.....\n#....\n#....\n#..#.\n##.##\n#####\n#####\n\n#####\n#####\n.##.#\n..#.#\n..#.#\n....#\n.....\n\n.....\n.....\n#..#.\n#.##.\n#.###\n#.###\n#####\n\n.....\n...#.\n...##\n#.###\n#.###\n#####\n#####\n\n#####\n#####\n.###.\n.#.#.\n...#.\n...#.\n.....\n\n.....\n.....\n.#.#.\n.#.#.\n##.##\n##.##\n#####\n\n.....\n...#.\n..##.\n..##.\n..##.\n.####\n#####\n\n.....\n.#...\n.#..#\n.#..#\n##..#\n##.##\n#####\n\n.....\n#.#..\n#.#..\n#.#..\n#.#.#\n###.#\n#####\n\n#####\n.###.\n.###.\n.###.\n.#.#.\n...#.\n.....\n\n#####\n#####\n.#.##\n.#.##\n.#.#.\n.#...\n.....\n\n.....\n.#...\n.#.#.\n.#.#.\n.#.#.\n.###.\n#####\n\n#####\n#.###\n#.###\n#.###\n..##.\n...#.\n.....\n\n.....\n.....\n.#...\n.#..#\n.#..#\n##.##\n#####\n\n.....\n..#..\n..#.#\n.##.#\n.##.#\n.##.#\n#####\n\n#####\n#####\n.#.##\n...##\n....#\n.....\n....."
  out "Answer 3508":u32
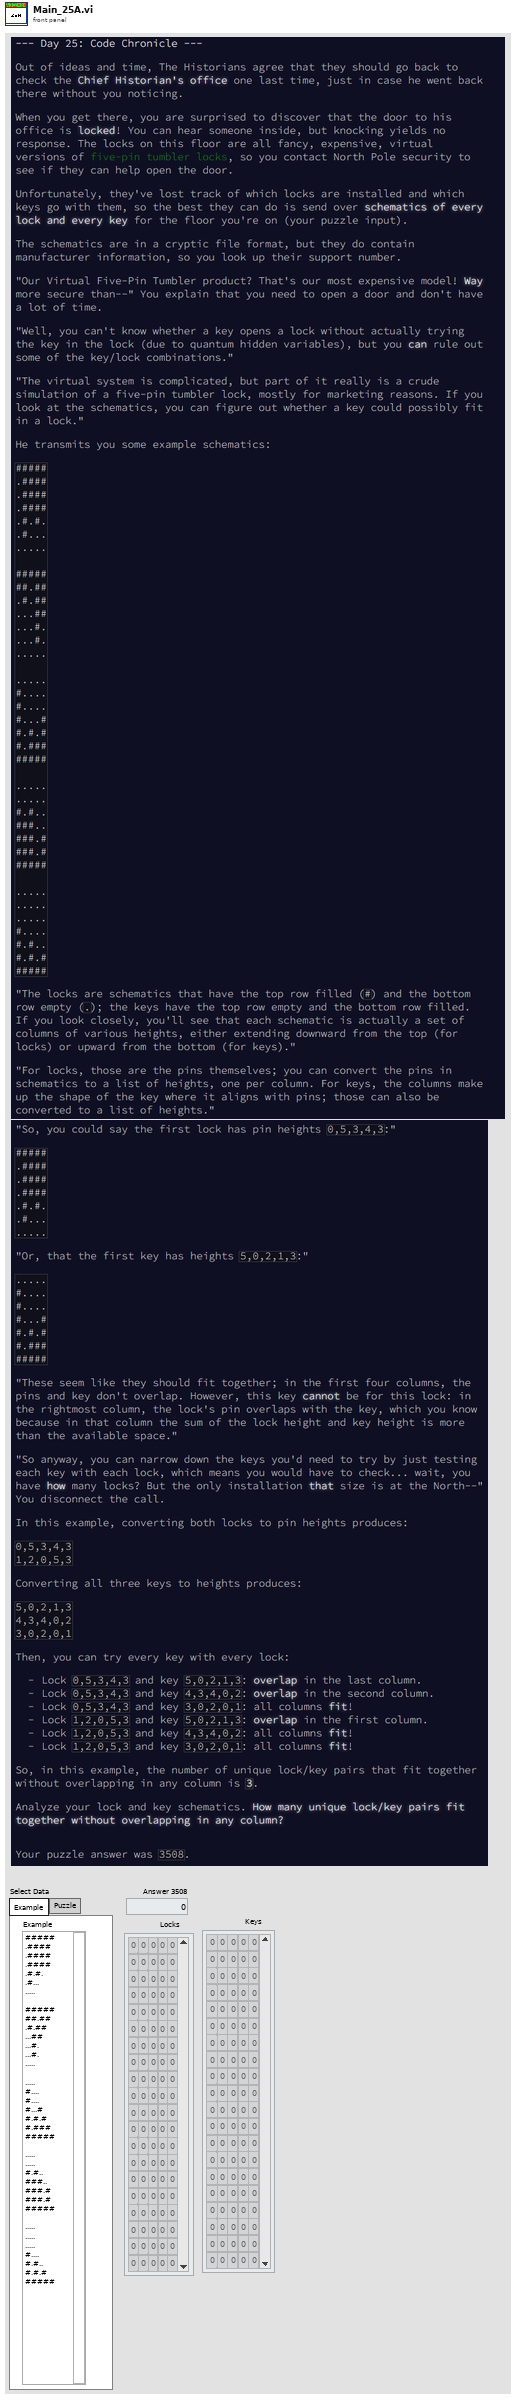
[diagram p1: front panel]
types:
  T1 = typedef "ENUM_8 Directions U-D-L-R.ctl" = enum16{"Up;-1,0", "Up-Right;-1,1", "Right;0,1", "Down-Right;1,1", "Down;1,0", "Down-Left;1,-1", "Left;0,-1", "Up-Left;-1,-1"}
  T2 = typedef "ENUM_4 Directions U-D-L-R.ctl" = enum16{"Up;-1,0", "Right;0,1", "Down;1,0", "Left;0,-1"}
  T3 = typedef "Cluster_Row-Column.ctl" = cluster{"R":i32, "C":i32}
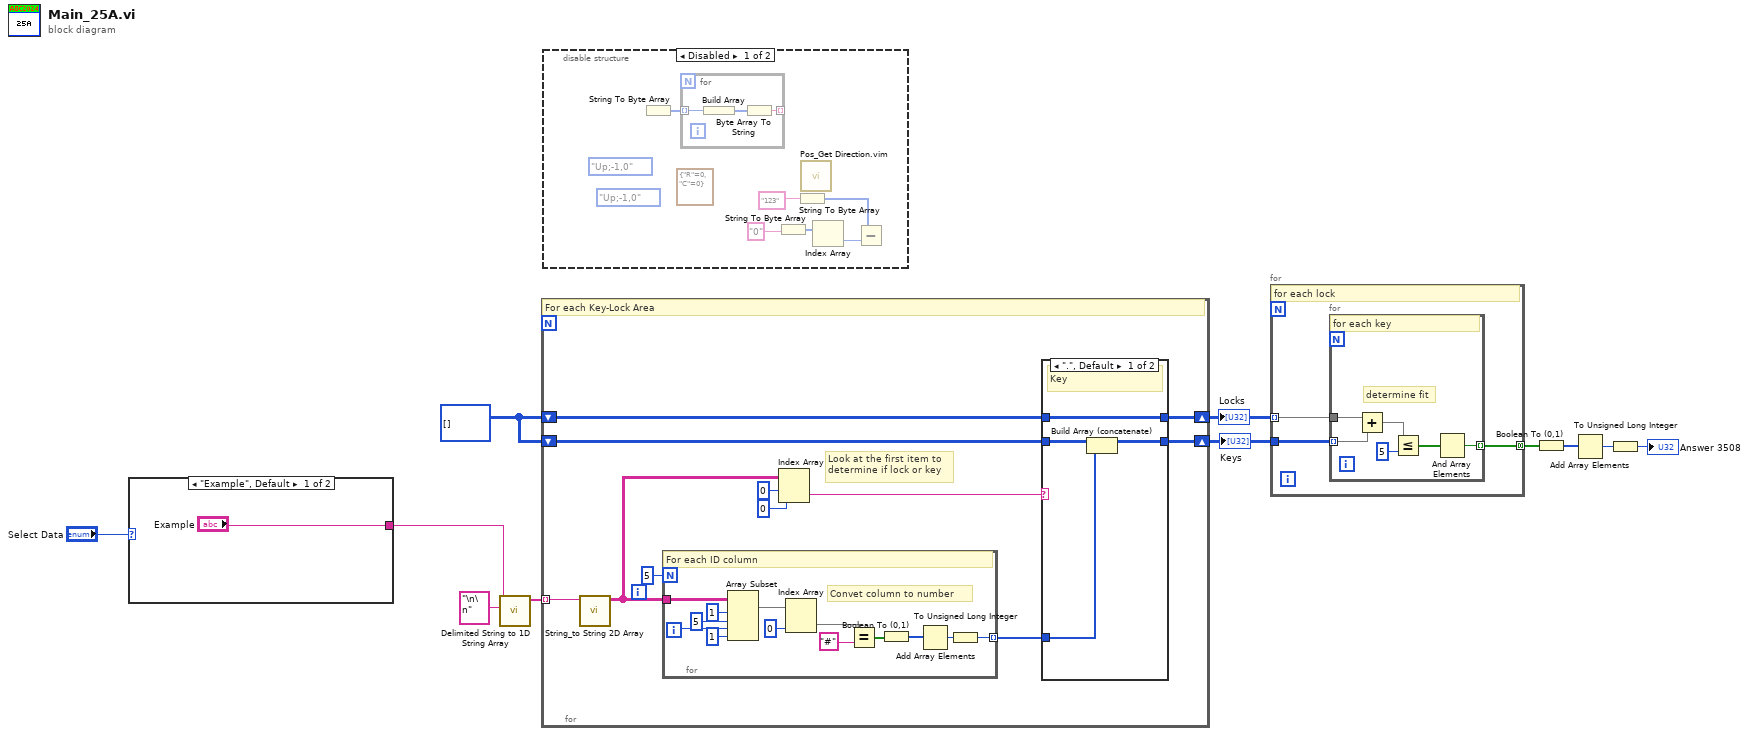
[diagram p0: block diagram]
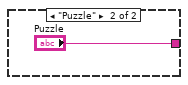
[diagram p2: hidden frame]
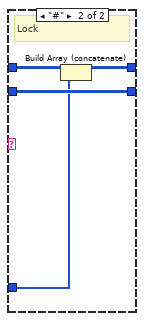
[diagram p4: hidden frame]
diagram:
  w7 = u32[][] []
  n1 = case shown="\"Example\", Default" "Select Data" {
    tunnel: ["Example" "Puzzle"] -> w8
    frame "Example", Default {
    }
    frame "Puzzle" {
    }
  }
  n2 = call <vilib>:"Delimited String to 1D String Array.vi"("delimiter"="\n\n" ("delimiter (Tab)"), "delimited string"=w8) -> ("string array"=w10:string[])  [unwired: 9 in]
  n3 = for {
    tunnel: w10 -> [w24] mode=indexing
    shift-right: [w14] -> w5
    shift-left: w7 -> [w18]
    shift-right: [w15] -> w6
    shift-left: w7 -> [w17]
    # "Look at the first item to\ndetermine if lock or key"
    # "For each Key-Lock Area"
    n4 = call "String_to String 2D Array.vi"("Input String"=w24) -> ("2D Array"=w23:string[][])  [unwired: 10 in]
    n5 = for {
      N: 5 -> [_]
      tunnel: w23 -> [w45]
      tunnel: [w33] -> w16 mode=indexing
      i -> [w37]
      # "Convet column to number"
      # "For each ID column"
      n6 = Array Subset(array=w45, index (row)=1 ("index"), length (row)=5 ("length"), index (col)=w37, length (col)=1 ("length")) -> (w41:string[][])
      n7 = Index Array(array=w41, index (col)=0 ("disabled index (col)")) -> (element=w39:string[])  [unwired: 1 in]
      n8 = Equal?(x=w39, y="#") -> (x = y?=w36:bool[])
      n9 = Boolean To (0,1)(Boolean=w36) -> (0, 1=w35:i16[])
      n10 = Add Array Elements(numeric array=w35) -> (sum=w34:i16)
      n11 = To Unsigned Long Integer(number=w34) -> (unsigned 32bit integer=w33:u32)
    }
    n12 = Index Array(array=w23, index (row)=0, index (col)=0 ("disabled index (col)")) -> (element=w19:string)
    n13 = case shown="\".\", Default" w19 {
      tunnel: w18 -> [w25 w31]
      tunnel: w17 -> [w28 w32]
      tunnel: w16 -> [w27 w29]
      tunnel: [w26 w32] -> w15
      tunnel: [w25 w30] -> w14
      frame ".", Default {
        # "Key"
        n14 = Build Array (concatenate)(w28, w27) -> (w26:u32[][])
      }
      frame "#" {
        # "Lock"
        n15 = Build Array (concatenate)(w31, w29) -> (w30:u32[][])
      }
    }
  }
  "Locks" <- w5
  "Keys" <- w6
  n16 = disable-structure shown="Disabled" {
    frame Disabled {
      (unwired) ENUM_8_Directions_U-D-L-R."Up;-1,0" ("Direction 8")
      (unwired) ENUM_4_Directions_U-D-L-R."Up;-1,0" ("Direction")
      (unwired) T3 {"R"=0, "C"=0} ("Position")
      n17 = String To Byte Array() -> (unsigned byte array=w46:u8[])  [unwired: 1 in]
      n18 = for {
        tunnel: w46 -> [w54] mode=indexing
        tunnel: [w52] -> _ mode=indexing
        n19 = Build Array(w54) -> (w53:u8[])
        n20 = Byte Array To String(unsigned byte array=w53) -> (string=w52:string)
      }
      n21 = String To Byte Array(string="0") -> (unsigned byte array=w49:u8[])
      n22 = String To Byte Array(string="123") -> (unsigned byte array=w47:u8[])
      n23 = call "Pos_Get Direction.vim"() -> ()  [unwired: 11 in, 1 out]
      n24 = Index Array(array=w49) -> (element=w48:u8)  [unwired: 1 in]
      n25 = Subtract(x=w47, y=w48) -> ()  [unwired: 1 out]
    }
    frame Enabled {
    }
  }
  n26 = for {
    tunnel: w6 -> [w57]
    tunnel: w5 -> [w56] mode=indexing
    tunnel: [w55] -> w3 mode=concatenating
    # "for each lock"
    n27 = for {
      tunnel: w57 -> [w62] mode=indexing
      tunnel: w56 -> [w63]
      tunnel: [w58] -> w55 mode=indexing
      # "determine fit"
      # "for each key"
      n28 = Add(x=w63, y=w62) -> (x+y=w61:u32[])
      n29 = Less Or Equal?(x=w61, y=u32 5 ("number")) -> (x <= y?=w59:bool[])
      n30 = And Array Elements(Boolean array=w59) -> (logical AND=w58:bool)
    }
  }
  n31 = Boolean To (0,1)(Boolean=w3) -> (0, 1=w4:i16[])
  n32 = Add Array Elements(numeric array=w4) -> (sum=w2:i16)
  n33 = To Unsigned Long Integer(number=w2) -> (unsigned 32bit integer=→"Answer 3508":u32)
